vi "FXP_Matrix-Vector_mult_loop_32bit.vi"(9 "Ns_2":u8=9, 11 "inputValid":bool) -> (2 "Array":fxp<+/-,32,13>[](array[numeric]))   [LabVIEW 2017]
doc: "Multiplies <B>Matrix A</B> by an input <B>Vector b</B>. This operation is useful for FPGA control applications, such as state-feedback control. You can use more than one multiplier to reduce the latency of this operation. To define <B>Matrix A</B>, double-click this Express VI and use the <B>Matrix Data Initialization</B> page to specify a VI, TXT, or CSV file that contains the matrix data. If you do not define <B>Matrix A</B>, this Express VI uses a matrix of zeroes instead.\n--------------------\n\nThis Express VI is configured as follows:\n\n<b>Fixed-Point Configuration</b>\nMatrix A Type: <+/-,32,16>\nVector b Type: <+/-,32,16>\nVector c Type: <+/-,64,36>\nOverflow mode: Truncate [Not Needed]\nRounding mode: Saturate [Not Needed]\n\n<b>Matrix A Configuration</b>\nMatrix Dimensions: 9 * 9\n\n<b>Multiplier Configuration</b>\nNumber of multipliers: 9\nNumber of multiplier pipeline stages: 0\n\n<b>Implementation</b>\nMatrix Vector Multiplication: 11 cycles"
uses:
  <vilib>/Platform/TimedLoop/XDataNode/timing_clust.ctl
  <vilib>/Platform/TimedLoop/XDataNode/nitl_modes.ctl
  <vilib>/Platform/TimedLoop/XDataNode/wakeup.ctl
  typeDefs/A_as_vec_bram.ctl
  typeDefs/x_vec_bram.ctl
  <vilib>/rvi/IPIntegrationNode/IPINode_Typedef/niFpgaIPINodeSupportedFamilies.ctl
  <vilib>/rvi/Emulation/niFpgaSctlEmulationGetInTimedLoop.vi
  <vilib>/rvi/Emulation/niFpgaEmulationReportErrorSimple.vi
  <vilib>/rvi/Emulation/niFpgaGetClockAttributes.vi
  <vilib>/rvi/Emulation/niFpgaCriticalErrorInLSC.vi
  <vilib>/rvi/IPIntegrationNode/IPINode_Utilities/niFpgaIPINodeSimCore.vi
  <vilib>/rvi/DataTransferAndStorage/Container/Common/niFpgaContainerExecOnDevCompGetState.vi
  <vilib>/rvi/Emulation/niFpgaEmulationIsFPGAContextNoSignature.vi
  <vilib>/rvi/DataTransferAndStorage/Container/Common/niFpgaContainerGetUniqueNameForEmu.vi
  <vilib>/rvi/Emulation/niFpgaProcessEmulError.vi
  <vilib>/rvi/errors/nirviReportUnexpectedCaseInternalError (U32).vi
  <vilib>/rvi/Memory/Memory_Emulation/niFpgaMemoryEmulationCacheClearOnFirstRun.vi
  <vilib>/rvi/Memory/Memory_Emulation/nirvimemoryEmulationManagerCache_MakeExclusive.vi
  <vilib>/rvi/Memory/Memory_Emulation/niFpgaMemoryEmulationValidateCache.vi
  <vilib>/rvi/Memory/Memory_Emulation/nirvimemoryEmulationManagerCache_InsertValue.vi
  <vilib>/Utility/error.llb/Clear Errors.vi
  <vilib>/rvi/Memory/Memory_Emulation/nirvimemoryEmulationManagerCache_ReleaseExclusive.vi
  <vilib>/rvi/Memory/Memory_Emulation/nirvimemoryEmulationManagerCache_GetValue.vi
  <vilib>/rvi/Memory/Memory_Emulation/nirvimemoryEmulationManagerCache_SetValue.vi
  <vilib>/rvi/Emulation/niFpgaSctlEmulationResourceMgr.vi
  <vilib>/Platform/TimedLoop/XDataNode/XDataNode.xnode
  <vilib>/rvi/XilinxIP/XIPIN_XNode/niFpgaXIPIN.xnode
  MAC01 1/MAC01_1_75F243352369479695E2AED5F4206BF1.dll
  <vilib>/rvi/IPIntegrationNode/IPINode_Xnode/niFpgaIPINode.xnode
  <vilib>/rvi/DataTransferAndStorage/Container/XNode/niFpgaContainer.xnode
  <vilib>/rvi/Memory/Memory_Emulation/niFpgaMemoryEmulationRefIn.vi
  <vilib>/Platform/TimedLoop/XDataNode/XDNodeRunTimeDep.lvlib
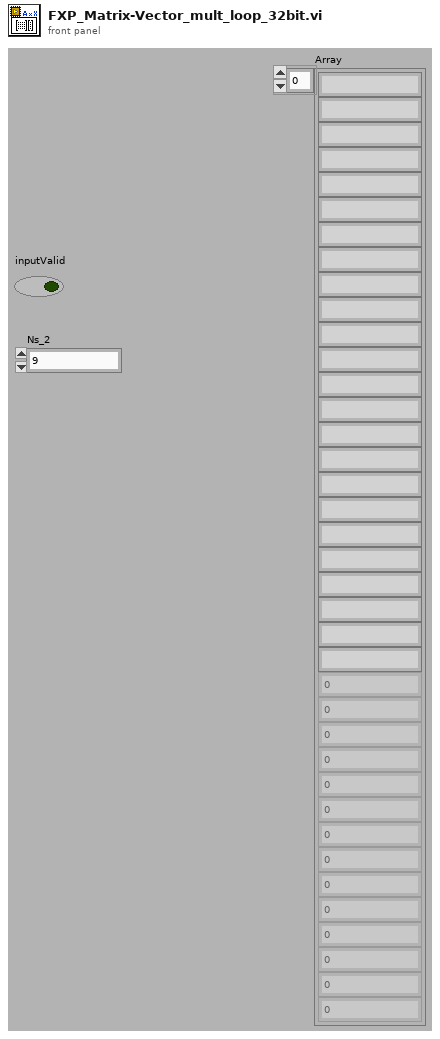
[diagram p1: front panel]
types:
  T1 = typedef "x_vec_bram.ctl" = refnum<k21>
  T2 = typedef "A_as_vec_bram.ctl" = refnum<k21>
  T3 = typedef "XDNodeRunTimeDep.lvlib/timing_clust.ctl" = cluster{"Expected End [f-1]":u64, "Actual End [f-1]":u64, "Finished Late? [f-1]":bool, "Expected End [i-1]":u64, "Actual End [i-1]":u64, "Finished Late? [i-1]":bool, "Expected Start [i]":u64, "Actual Start [i]":u64, "Expected Start [f]":u64, "Actual Start [f]":u64, "Source Name":string, "Structure Name":string, "Period":i64, "Deadline":i64, "Offset":i64, "Start":i64, "Priority":i32, "Timeout":i32, "Mode":T4, "Wakeup Reason":T5, "Error":errorcluster, "Source Type":string, "Secondary Source Type":string, "Global End Time":u64, "Global Start Time":u64, "Frame Duration":u64, "Iteration Duration":u64, "Assigned CPU":i32, "I/O Scan Engine Mode":u32}
  T4 = typedef "XDNodeRunTimeDep.lvlib/nitl_modes.ctl" = enum32{"No Change", "Process missed periods, maintain original phase", "Discard missed periods, maintain original phase", "Process missed periods, ignore original phase", "Discard missed periods, ignore original phase"}
  T5 = typedef "XDNodeRunTimeDep.lvlib/wakeup.ctl" = enum32{"Normal", "Aborted", "Asynchronous wakeup", "Timing source error", "Timed loop error", "Timeout"}
  T6 = typedef "niFpgaIPINodeSupportedFamilies.ctl" = cluster{"unlimited?":bool, "supported targets":string[]}
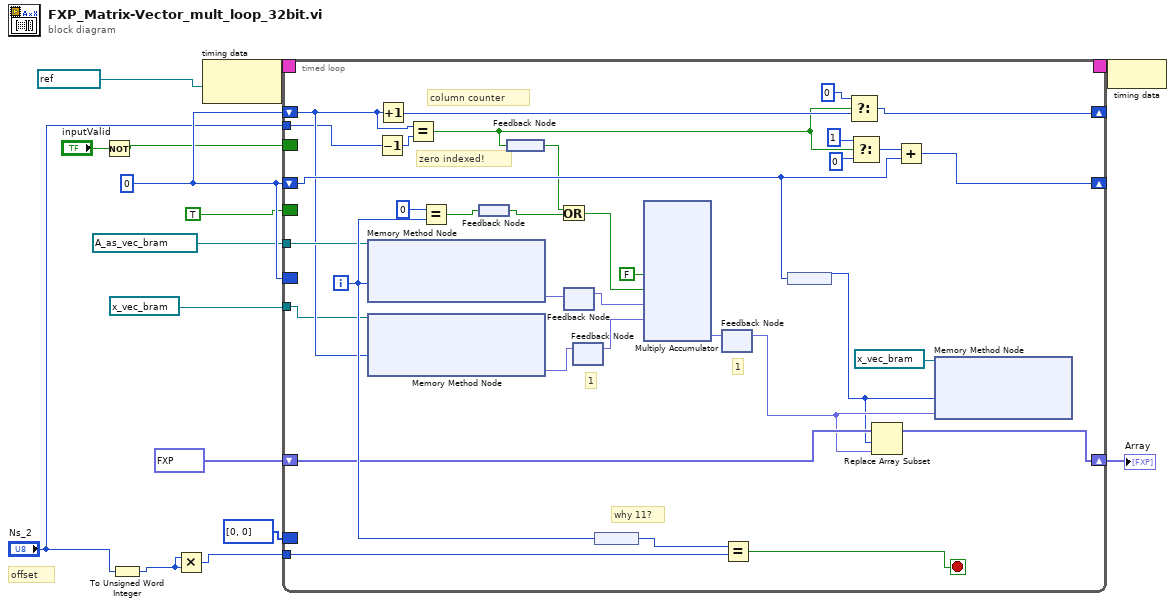
[diagram p0: block diagram]
diagram:
  w13 = u8 0
  # "offset"
  n1 = Not(x="inputValid") -> (.not. x?=w10:bool)
  n2 = To Unsigned Word Integer(number="Ns_2") -> (unsigned 16bit integer=w12:u16)
  n3 = Multiply(x=w12, y=w12) -> (x*y=w5:u16)
  n4 = node-c288(refnum<k21> "80MHz" ("Source Name")) -> (w15:T3)
  n5 = timed-loop {
    timing: w15 -> [_]
    timing-out: [_] -> w14
    shift-right: [w44] -> _
    shift-left: w13 -> [w41]
    shift-right: [w48] -> _
    shift-left: w13 -> [w30]
    border: w10 -> [_]
    border: w13 -> [_]
    tunnel: T2 "AasCol _FXP" ("Memory In") -> [w32]
    tunnel: w5 -> [w31]
    tunnel: T1 "xk_1_1" ("Memory") -> [w29]
    shift-right: [w27] -> w7
    shift-left: fxp<+/-,32,13>[] [0.0, 0.0, 0.0, 0.0, 0.0, 0.0, 0.0, 0.0, 0.0, 0.0, 0.0, 0.0, 0.0, 0.0, 0.0, 0.0, 0.0, 0.0, 0.0, 0.0, 0.0, 0.0, 0.0, 0.0] ("Array 2") -> [w28]
    border: TRUE -> [_]
    border: i32[] [0, 0] -> [_]
    tunnel: "Ns_2" -> [w24]
    i -> [w34]
    stop <- w49 stop-if-true
    # "why 11?"
    # "1"
    # "1"
    # "zero indexed!"
    # "column counter"
    n6 = xnode ("Memory Method Node")("Address"=w34, "Memory In"=w32) -> ("Data"=w23:fxp<+/-,32,7>)  [unwired: 1 out]
    n7 = xnode ("Memory Method Node")("Address"=w30, "Memory In"=w29) -> ("Data"=w20:fxp<+/-,32,6>)  [unwired: 1 out]
    n8 = Decrement(x=w24) -> (x-1=w39:u8)
    n9 = Increment(x=w30) -> (x+1=w43:u8)
    n10 = Equal?(x=w30, y=w39) -> (x = y?=w40:bool)
    n11 = Equal?(x=0, y=w34) -> (x = y?=w25:bool)
    n12 = feedback #1() -> (w26:bool)
    n13 = feedback-in #1(w25) -> ()
    n14 = feedback #2() -> (w38:bool)
    n15 = feedback-in #2(w40) -> ()
    n16 = Or(x=w38, y=w26) -> (x .or. y?=w37:bool)
    n17 = feedback-in #3(w23) -> ()
    n18 = feedback #3() -> (w22:fxp<+/-,32,7>)  [unwired: 1 in]
    n19 = feedback #4() -> (w21:fxp<+/-,32,6>)  [unwired: 1 in]
    n20 = feedback-in #4(w20) -> ()
    n21 = feedback #5() -> (w35:i32)
    n22 = feedback-in #5(w34) -> ()
    n23 = xnode ("Multiply Accumulator")("sclr"=FALSE, "bypass"=w37, "a"=w22, "b"=w21) -> ("s"=w19:fxp<+/-,36,13>)  [unwired: 1 in]
    n24 = feedback #6() -> (w17:fxp<+/-,36,13>)  [unwired: 1 in]
    n25 = feedback-in #6(w19) -> ()
    n26 = Equal?(x=w35, y=w31) -> (x = y?=w49:bool)
    n27 = feedback #7() -> (w16:u8)
    n28 = feedback-in #7(w41) -> ()
    n29 = Select(t=u8 0, s=w40, f=w43) -> (s? t:f=w48:u8)
    n30 = Select(t=u8 1, s=w40, f=u8 0) -> (s? t:f=w45:u8)
    n31 = Replace Array Subset(array=w28, new element=w17, index=w16) -> (w27:fxp<+/-,32,13>[])
    n32 = Add(x=w45, y=w41) -> (x+y=w44:u8)
    n33 = xnode ("Memory Method Node")("Address"=w16, "Data"=w17, "Memory In"=T1 "xk_1_0" ("Memory")) -> ()  [unwired: 1 out]
  }
  "Array" <- w7
  n34 = node-c288(w14) -> ()
